vi "Create Test Configuration.vi"() -> (0 "error out":errorcluster, 1 "Names":string[](array[string]), 2 "Line Array":T1[](array[typedef]), 3 "Module Configuration":refnum<class "SQLite configuration.lvclass">, 4 "Channels":refnum<class "TBM channel.lvclass">[](array[class]), 5 "instance identifier":string)   [LabVIEW 2014, in "SQLite tests.lvlib"]
doc: "This VI creates a standard test configuration for other unit tests. It currently creates and adds one line with every datatype to the module configuration."
uses:
  SQLite tests.lvlib
  module/configuration/SQLite configuration.lvclass
  module/configuration/Line.ctl
  <vilib>/NI/Tag Bus Module Framework/channel/TBM channel.lvclass
  <vilib>/NI/Tag Bus Module Framework/channel/channel classification.ctl
  <vilib>/NI/Configuration Framework/serializable configuration/NISE_CEF_serializable configuration.lvclass
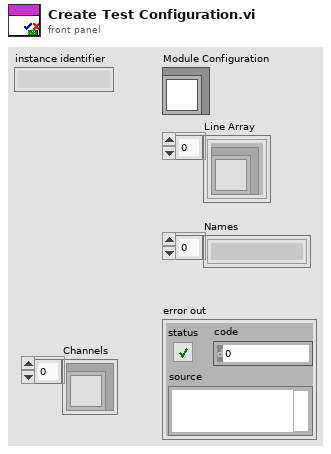
[diagram p1: front panel]
types:
  T1 = typedef "SQLite configuration.lvclass/Line.ctl" = cluster{"channel":refnum<class "TBM channel.lvclass">}
  T2 = typedef "TBM channel.lvclass/channel classification.ctl" = enum16{"input data", "output data", "processing parameter", "processing result"}
  T3 = typedef "tag bus.lvlib/tag descriptor.lvclass/Data Type.ctl" = enum16{"Double", "Single", "I64", "I32", "I16", "I8", "U64", "U32", "U16", "U8", "Boolean", "String", "Array of Double", "Array of Single", "Array of I64", "Array of I32", "Array of I16", "Array of I8", "Array of U64", "Array of U32", "Array of U16", "Array of U8", "Array of Boolean", "Array of String"}
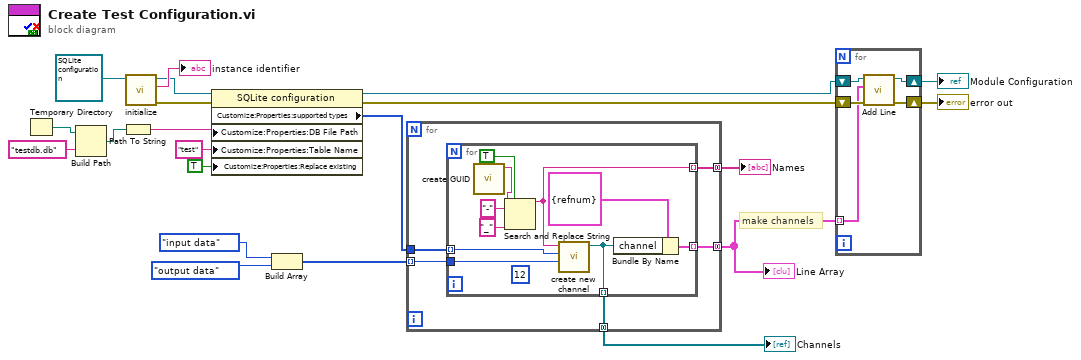
[diagram p0: block diagram]
diagram:
  # "make channels"
  n1 = Temporary Directory() -> (w4:path)
  n2 = Build Path(base path=w4, name or relative path="testdb.db") -> (appended path=w3:path)
  n3 = Path To String(path=w3) -> (string=w2:string)
  n4 = call <vilib>:"initialize.vi"("configuration in"=refnum<class "SQLite configuration.lvclass"> refnum ("tag bus configurable plugin module configuration")) -> ("error out"=w19:errorcluster, "identifier"=→"instance identifier":string, "configuration out"=w16:refnum<class "SQLite configuration.lvclass">)  [unwired: 8 in]
  n5 = property class="SQLite configuration"(reference=w16, error in=w19, "Customize:Properties:DB File Path"=w2, "Customize:Properties:Table Name"="test" ("Table Name"), "Customize:Properties:Replace existing"=TRUE ("Replace existing")) -> (reference out=w11:refnum<class "SQLite configuration.lvclass">, error out=w18:errorcluster, "Customize:Properties:supported types"=w12:T3[])
  n6 = Build Array(channel_classification."input data" ("channel classification"), channel_classification."output data" ("channel classification")) -> (w10:T2[])
  n7 = for {
    tunnel: w10 -> [w26] mode=indexing
    tunnel: [w24] -> w15 mode=concatenating
    tunnel: w12 -> [w25]
    tunnel: [w23] -> w17 mode=concatenating
    tunnel: [w22] -> w7 mode=concatenating
    n8 = for {
      tunnel: w26 -> [w36]
      tunnel: [w33] -> w24 mode=indexing
      tunnel: w25 -> [w35] mode=indexing
      tunnel: [w30] -> w23 mode=indexing
      tunnel: [w32] -> w22 mode=indexing
      (unwired) 12
      n9 = call <vilib>:"create GUID.vi"() -> ("uuid"=w31:string)  [unwired: 10 in, 1 out]
      n10 = Search and Replace String(replace all?=TRUE ("replace all? (F)"), input string=w31, search string="-", replace string="_" ("replace string (\"\")")) -> (result string=w30:string)  [unwired: 4 in, 3 out]
      n11 = call <vilib>:"create new channel.vi"("channel classification"=w36, "data type"=w35, "channel name"=w30) -> ("channel"=w32:refnum<class "TBM channel.lvclass">)  [unwired: 8 in]
      n12 = Bundle By Name(cluster=T1 {"channel"=refnum} ("Line"), "channel"=w32) -> (w33:T1)
    }
  }
  "Names" <- w17
  "Line Array" <- w15
  "Channels" <- w7
  n13 = for {
    tunnel: w15 -> [w37] mode=indexing
    shift-right: [w40] -> w14
    shift-left: w11 -> [w41]
    shift-right: [w38] -> w21
    shift-left: w18 -> [w39]
    n14 = call "Add Line.vi"("error in"=w39, "Line"=w37, "SQLite configuration in"=w41) -> ("error out"=w38:errorcluster, "SQLite configuration out"=w40:refnum<class "SQLite configuration.lvclass">)  [unwired: 6 in, 1 out]
  }
  "error out" <- w21
  "Module Configuration" <- w14
